vi "iToTime.vi"(2 "Error In":errorcluster, 3 "time":dbl[](array[numeric]), 4 "iArray":dbl[](array[numeric])) -> (0 "Error Out":errorcluster, 1 "timeArray":dbl[](array[numeric]))   [LabVIEW 2015]
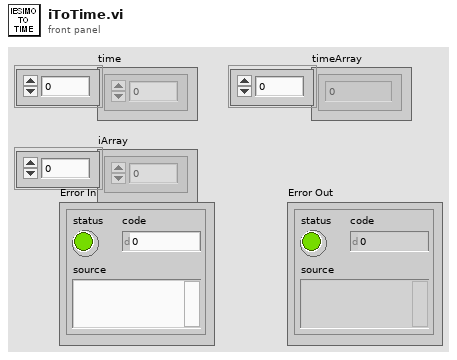
[diagram p1: front panel]
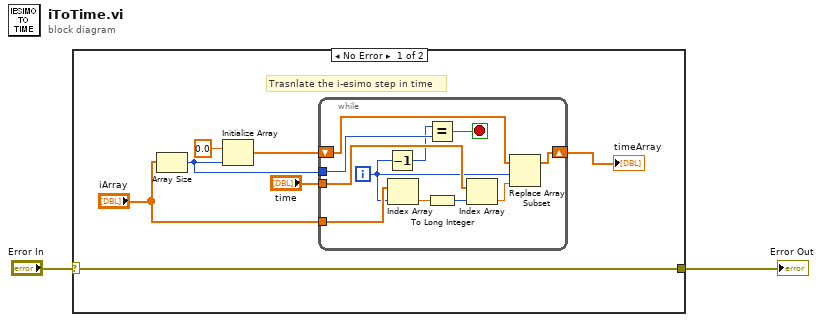
[diagram p0: block diagram]
diagram:
  n1 = case shown="No Error" "Error In" {
    selector: "Error In" -> [w3 w21]
    tunnel: [w3 w21] -> w1
    frame No Error {
      # "Trasnlate the i-esimo step in time"
      n2 = Array Size(array="iArray") -> (size(s)=w7:i32)
      n3 = Initialize Array(0.0 ("element"), w7) -> (w4:dbl[])
      n4 = while {
        tunnel: "iArray" -> [w20]
        tunnel: "time" -> [w18]
        tunnel: w7 -> [w12]
        shift-right: [w15] -> w9
        shift-left: w4 -> [w16]
        i -> [w13]
        stop <- w11 stop-if-true
        n5 = Decrement(x=w13) -> (x-1=w10:i32)
        n6 = Index Array(array=w20, index=w13) -> (element=w19:dbl)
        n7 = Equal?(x=w10, y=w12) -> (x = y?=w11:bool)
        n8 = To Long Integer(number=w19) -> (32bit integer=w17:i32)
        n9 = Index Array(array=w18, index=w17) -> (element=w14:dbl)
        n10 = Replace Array Subset(array=w16, new element=w14, index=w13) -> (w15:dbl[])
      }
      "timeArray" <- w9
    }
    frame Error {
    }
  }
  "Error Out" <- w1
